vi "Stepper Sequence Change Focus.vi"() -> ()   [LabVIEW 2013]
doc: "Writes specified digital values to all 14 digital I/O pins. Each pin must first be configured as a digital output using the Arduino Set Digital Pin Mode VI."
uses:
  Hello Optotune Lens (30.06.2014)/Calibration.ctl
  <vilib>/Math Plots/3D Math Plots/3D Surface/3D Surface XCtrl/3D Surface.xctl
  <vilib>/LabVIEW Interface for Arduino/Type Defs/Board Type.ctl
  <vilib>/LabVIEW Interface for Arduino/Type Defs/Analog Pin.ctl
  <vilib>/Instr/_visa.llb/VISA Configure Serial Port (Instr).vi
  <vilib>/Math Plots/3D Math Plots/3D Surface/3D Surface Datatype/Public/Plot Helper (Matrix).vi
  <vilib>/LabVIEW Interface for Arduino/LabVIEW Interface for Arduino.lvlib
  <vilib>/Math Plots/3D Math Plots/3D Surface/3D Surface Datatype/3D Surface Datatype.lvclass
panel:
  out "3D Surface":refnum<class "3D Plot Datatype.lvclass">[](xcontrol)
  in  "Anahl Messungen":i32
  out "Aktuelle Messung":i32
  in  "Maximaler Strom":dbl=290.0
  out "Array 2":dbl[](array[numeric])
  out "Voltage 2":dbl(knob)=0.0294 scale=0.0..5.0
  in  "Stepwidth X":dbl=20.0
  out "Array":dbl[](array[numeric])=[0.0784, 0.0, 0.0, 0.0, 0.049, 0.053899999999999997, 0.0784, 0.0392, 0.0588, 0.0294]
  out "Aktueller Linsenstrom":dbl=49.0
  out "Schritt 7":bool
  out "Schritt 6":bool
  out "Schritt 5":bool
  out "Schritt 4":bool
  out "Schritt 3":bool
  out "Schritt 2":bool
  out "Schritt 1":bool=TRUE
  out "Value":u8
  out "x = y?":bool=TRUE
  in  "STOP INTIAL":bool
  out "VISA resource name out 3":refnum<visa-resource-name>="COM13"
  out "Command to Port 2":string="Aw\n´"
  out "Number of Measurements":i8=6
  in  "Min Focal Length 2":dbl
  in  "Max Focal Length":dbl=293.0
  out "Position_aktuell":dbl=90.0
  in  "First Motor Pin":u8=3
  in  "Pin Endlagenschalter":u8=32
  in  "Stepwidth Focalwidth lens":dbl=50.0
  in  "Calibration":T1={"Max Current A"=293.0, "Max Current B"=293.0, "UCL A"=300.0, "UCL B"=300.0, "LCL A"=0.0, "LCL B"=0.0} {"Max Current A" format="%#_g mA"; "Max Current B" format="%#_g mA"; "UCL A" format="%#_g mA"; "LCL A" format="%#_g mA"; "UCL B" format="%#_g mA"; "LCL B" format="%#_g mA"}
  out "ID":u16
  out "VISA resource name out":string="COM13"
  out "Calibration 2":T1={"Max Current A"=292.84, "Max Current B"=293.0, "UCL A"=292.76850585937495, "UCL B"=300.0, "LCL A"=4392.671494140624, "LCL B"=0.0} {"Max Current A" format="%#_g mA"; "Max Current B" format="%#_g mA"; "UCL A" format="%#_g mA"; "LCL A" format="%#_g mA"; "UCL B" format="%#_g mA"; "LCL B" format="%#_g mA"}
  out "OK":bool=TRUE
  out "Data":string
  out "Command to Port":string
  out "TA (°C)":dbl=32.125
  out "error out":errorcluster={"status"=FALSE, "code"=1073676294, "source"="VISA Read in write read Lens Driver.vi->Stepper Sequence Change Focus.vi"}
  in  "error in (no error)":errorcluster
  in  "VISA resource name":string="COM13"
  in  "Initial Speed":dbl=1.0
  # "Lens Settings"
  # "Measurement Settings"
  # "Initial Settings"
  # "mA"
  # "0 Fast, 100 slow"
  # "mA"
  # "Diodenstrom I0"
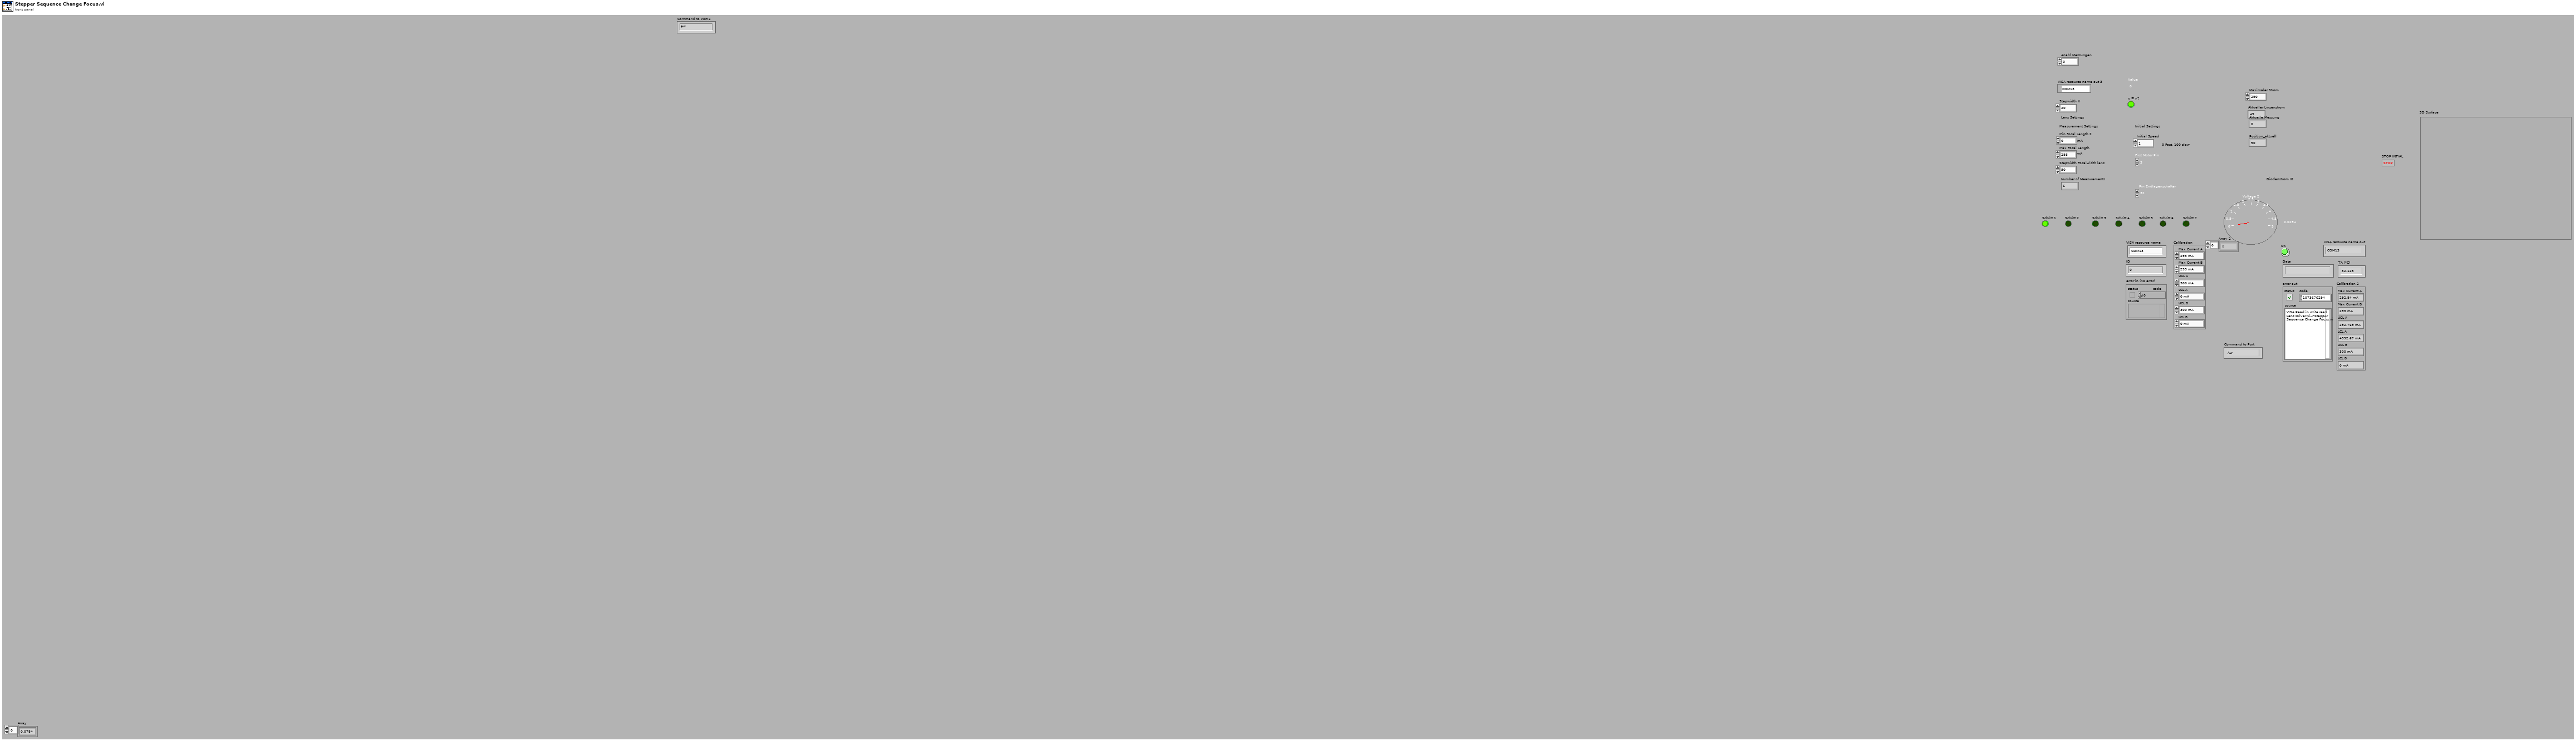
[diagram p1: front panel]
types:
  T1 = typedef "Calibration.ctl" = cluster{"Max Current A":dbl, "Max Current B":dbl, "UCL A":dbl, "UCL B":dbl, "LCL A":dbl, "LCL B":dbl}
  T2 = typedef "LabVIEW Interface for Arduino.lvlib/Board Type.ctl" = enum16{"Uno", "Dimuelanove w/Atmega 328", "Mega 2560"}
  T3 = typedef "LabVIEW Interface for Arduino.lvlib/Arduino Resource.ctl" = cluster{"VISA resource":refnum<visa-resource-name>, "Board Type":T2, "Connection Type":enum8{"USB / Serial"}, "Bytes Per Packet (15)":u8}
  T4 = typedef "LabVIEW Interface for Arduino.lvlib/Analog Pin.ctl" = enum8{"Anlog In 0", "Anlog In 1", "Anlog In 2", "Anlog In 3", "Anlog In 4", "Anlog In 5"}
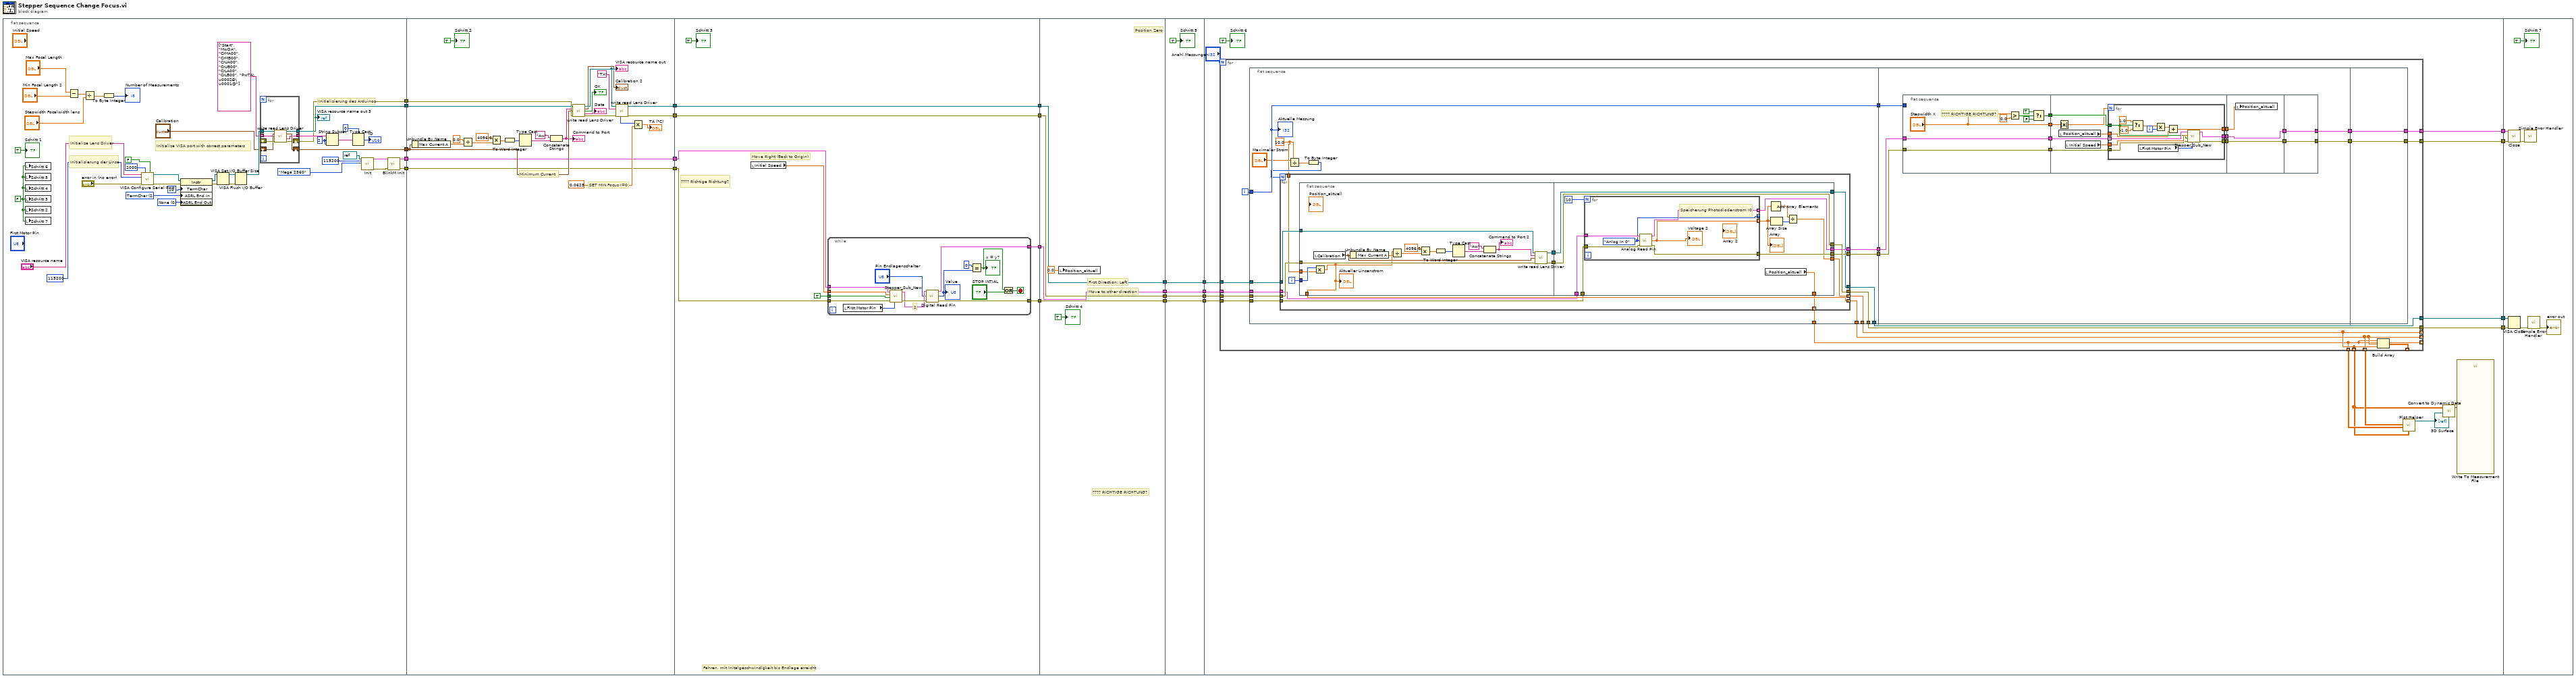
[diagram p0: block diagram]
diagram:
  n1 = flat-sequence {
    tunnel: [w43] -> w15
    tunnel: [w42] -> w14
    tunnel: [w41] -> w13
    tunnel: [w36] -> w5
    tunnel: [w35] -> w4
    tunnel: [w77] -> w25
    tunnel: [w76] -> w24
    tunnel: w15 -> [w99]
    tunnel: w14 -> [w98]
    tunnel: w13 -> [w97]
    tunnel: [w94] -> w12
    tunnel: [w78] -> w6
    tunnel: w5 -> [w77]
    tunnel: w4 -> [w76]
    tunnel: [w107] -> w19
    tunnel: w25 -> [w105]
    tunnel: [w106] -> w17
    tunnel: w24 -> [w108]
    tunnel: w12 -> [w104]
    tunnel: [w104] -> w11
    tunnel: [w103] -> w7
    tunnel: w6 -> [w103]
    tunnel: w19 -> [w129]
    tunnel: [w129] -> w18
    tunnel: w17 -> [w128]
    tunnel: [w128] -> w16
    tunnel: w11 -> [w127]
    tunnel: [w127] -> w10
    tunnel: [w126] -> w8
    tunnel: w7 -> [w126]
    tunnel: w18 -> [w133]
    tunnel: [w133] -> w23
    tunnel: w16 -> [w130]
    tunnel: [w130] -> w22
    tunnel: w10 -> [w132]
    tunnel: w8 -> [w131]
    tunnel: [w132] -> w3
    tunnel: [w131] -> w2
    tunnel: w23 -> [w149]
    tunnel: w22 -> [w148]
    tunnel: [w147] -> w21
    tunnel: [w146] -> w20
    tunnel: [w144] -> w9
    tunnel: w3 -> [w145]
    tunnel: w2 -> [w143]
    tunnel: [w141] -> w1
    tunnel: w21 -> [w290]
    tunnel: w20 -> [w289]
    tunnel: w9 -> [w286]
    tunnel: w1 -> [w287]
    frame #0 {
      w27 = FALSE ("Schritt 6")
      w63 = 2 ("length (rest)")
      w48 = u16 0 items=["None", "Last Bit", "TermChar", "Break"] ("Serial Settings:End Mode for Writes")
      w49 = u16 2 items=["None", "Last Bit", "TermChar"] ("Serial Settings:End Mode for Reads")
      # "Initialisierung des Arduinos"
      # "Initialisierung der Linse"
      # "Initialize Lens Driver"
      # "Initialize VISA port with correct parameters"
      n2 = local write "Schritt 6"(w27) -> ()
      n3 = local write "Schritt 5"(w27) -> ()
      n4 = local write "Schritt 4"(w27) -> ()
      n5 = local write "Schritt 3"(w27) -> ()
      n6 = local write "Schritt 2"(w27) -> ()
      n7 = local write "Schritt 7"(w27) -> ()
      n8 = Subtract(x="Max Focal Length", y="Min Focal Length 2") -> (x-y=w32:dbl)
      n9 = Divide(x=w32, y="Stepwidth Focalwidth lens") -> (x/y=w30:dbl)
      n10 = To Byte Integer(number=w30) -> (8bit integer=→"Number of Measurements":i8)
      n11 = call-poly "VISA Configure Serial Port"("VISA resource name"="VISA resource name", "timeout (10sec)"=u32 2000, "Enable Termination\nChar (T)"=FALSE ("Enable Termination\nChar (T)"), "baud rate (9600)"=u32 115200, "error in (no error)"="error in (no error)") -> ("VISA resource name out"=w53:refnum<visa-resource-name>, "error out"=w51:errorcluster)  [unwired: 9 in]
      n12 = property class="Instr"(reference=w53, error in=w51, "TermChar"=u8 10 ("Message Based Settings:Termination Character"), "ASRL End In"=w49, "ASRL End Out"=w48) -> (reference out=w52:refnum<visa-resource-name>, error out=w50:errorcluster)
      n13 = VISA Set I/O Buffer Size(VISA resource name=w52, error in (no error)=w50) -> (VISA resource name out=w45:refnum<visa-resource-name>, error out=w44:errorcluster)  [unwired: 2 in]
      n14 = VISA Flush I/O Buffer(VISA resource name=w45, error in (no error)=w44) -> (VISA resource name out=w65:refnum<visa-resource-name>)  [unwired: 1 in, 1 out]
      n15 = for {
        tunnel: w65 -> [w72]
        tunnel: [w69] -> w43
        tunnel: string[] ["Start", "MwDA", "CrMA00", "CrMB00", "CrUA00", "CrUB00", "CrLA00", "CrLB00", "PwTA\u0002Ð\u0001@"] -> [w67] mode=indexing
        tunnel: [w66] -> w59
        shift-right: [w70] -> w42
        shift-left: "Calibration" -> [w71]
        shift-right: [w68] -> w41
        shift-left: _ -> [w73]
        n16 = call "write read Lens Driver.vi"("VISA resource name"=w72, "command"=w67, "Calibration"=w71, "error in (no error)"=w73) -> ("VISA resource name out"=w69:refnum<visa-resource-name>, "Calibration 2"=w70:T1, "Data"=w66:string, "error out"=w68:errorcluster)  [unwired: 4 in, 4 out]
      }
      "VISA resource name out 3" <- w43
      n17 = String Subset(string=w59, offset (0)=w63, length (rest)=w63) -> (substring=w61:string)
      n18 = Type Cast(type=u16 0 ("length (rest)"), x=w61) -> (*(type *) &x=→"ID":u16)
      n19 = call <vilib>:"Init.vi"("VISA resource"=refnum<visa-resource-name> refnum, "Baud Rate (115200)"=u32 115200, "Board Type (Uno)"=Board_Type."Mega 2560") -> ("Arduino Resource"=w39:T3, "error out"=w40:errorcluster)  [unwired: 15 in]
      n20 = call <vilib>:"BlinkM Init.vi"("Arduino Resource"=w39, "error in"=w40) -> ("Arduino Resource"=w36:T3, "error out"=w35:errorcluster)  [unwired: 12 in]
      "Schritt 1" <- TRUE
    }
    frame #1 {
      # "Minimum Current"
      # "SET MIN Focus I=0"
      n21 = Unbundle By Name(w98) -> ("Max Current A"=w83:dbl)
      n22 = Divide(x=0.0, y=w83) -> (x/y=w90:dbl)
      n23 = Multiply(x=4096.0, y=w90) -> (x*y=w88:dbl)
      n24 = To Word Integer(number=w88) -> (16bit integer=w87:i16)
      n25 = Type Cast(x=w87) -> (*(type *) &x=w86:string)  [unwired: 1 in]
      n26 = Concatenate Strings("Aw", w86) -> (w84:string)
      "Command to Port" <- w84
      n27 = call "write read Lens Driver.vi"("VISA resource name"=w99, "command"=w84, "Calibration"=w98, "error in (no error)"=w97) -> ("VISA resource name out"=w96:refnum<visa-resource-name>, "Calibration 2"=→"Calibration 2":T1, "OK"=→"OK":bool, "Data"=→"Data":string, "error out"=w95:errorcluster)  [unwired: 4 in, 3 out]
      "VISA resource name out" <- w96
      n28 = call "write read Lens Driver.vi"("VISA resource name"=w96, "command"="TA", "error in (no error)"=w95) -> ("VISA resource name out"=w94:refnum<visa-resource-name>, "TA"=w80:u16, "error out"=w78:errorcluster)  [unwired: 5 in, 5 out]
      n29 = Multiply(x=w80, y=0.0625) -> (x*y=→"TA (°C)":dbl)
      "Schritt 2" <- TRUE
    }
    frame #2 {
      # "???? Richtige Richtung?"
      # "Move Right (Back to Origin)"
      # "Fahren, mit Initalgeschwindigkeit bis Endlage erreicht"
      n30 = local read "Initial Speed"() -> (w102:dbl)
      n31 = while {
        tunnel: w105 -> [w122]
        tunnel: w108 -> [w121]
        tunnel: TRUE -> [w119]
        tunnel: w102 -> [w120]
        tunnel: [w114] -> w107
        tunnel: [w113] -> w106
        stop <- w116 stop-if-true
        # "2"
        n32 = local read "First Motor Pin"() -> (w118:u8)
        n33 = call "Stepper_Sub_New.vi"("First Motor Pin"=w118, "error in"=w121, "Direction"=w119, "Velocity"=w120, "Arduino Resource"=w122) -> ("error out"=w111:errorcluster, "Arduino Resource 2"=w110:T3)  [unwired: 5 in]
        n34 = call <vilib>:"Digital Read Pin.vi"("Arduino Resource"=w110, "Digital I/O Pin (0)"="Pin Endlagenschalter", "error in"=w111) -> ("Arduino Resource"=w114:T3, "Value"=w112:u8, "error out"=w113:errorcluster)  [unwired: 10 in]
        "Value" <- w112
        n35 = Equal?(x=u8 0, y=w112) -> (x = y?=w117:bool)
        "x = y?" <- w117
        n36 = Or(x=w117, y="STOP INTIAL") -> (x .or. y?=w116:bool)
      }
      "Schritt 3" <- TRUE
    }
    frame #3 {
      # "???? RICHTIGE RICHTUNG?"
      # "Move to other direction"
      # "First Direction: Left"
      # "Position Zero"
      n37 = local write "Position_aktuell"(0.0 ("Position_aktuell")) -> ()
      "Schritt 4" <- TRUE
    }
    frame #4 {
      "Schritt 5" <- TRUE
    }
    frame #5 {
      n38 = for {
        N: "Anahl Messungen" -> [_]
        tunnel: w149 -> [w167]
        tunnel: w148 -> [w166]
        tunnel: [w165] -> w147
        tunnel: [w164] -> w146
        tunnel: w145 -> [w162]
        tunnel: w143 -> [w161]
        tunnel: [w159] -> w144
        tunnel: [w151] -> _ mode=indexing
        tunnel: [w155] -> w141
        tunnel: [w152] -> _ mode=indexing
        tunnel: [w150] -> _ mode=indexing
        tunnel: [w153] -> _ mode=indexing
        tunnel: [w152] -> w136 mode=indexing
        tunnel: [w151] -> w138 mode=indexing
        tunnel: [w150] -> w137 mode=indexing
        i -> [w160]
        n39 = flat-sequence {
          tunnel: w167 -> [w179]
          tunnel: w166 -> [w177]
          tunnel: [w178] -> w163
          tunnel: w162 -> [w183]
          tunnel: w161 -> [w180]
          tunnel: w160 -> [w173]
          tunnel: [w182] -> w159
          tunnel: [w181] -> w151
          tunnel: [w176] -> w156
          tunnel: [w175] -> w155
          tunnel: [w174] -> w152
          tunnel: [w173] -> w154
          tunnel: [w169] -> w150
          tunnel: w163 -> [w246]
          tunnel: [w245] -> w158
          tunnel: [w244] -> w157
          tunnel: w156 -> [w243]
          tunnel: w154 -> [w242]
          tunnel: [w284] -> w164
          tunnel: [w285] -> w165
          tunnel: w158 -> [w285]
          tunnel: w157 -> [w284]
          frame #0 {
            w168 = 10.0 ("y")
            n40 = Divide(x="Maximaler Strom", y=w168) -> (x/y=w171:dbl)
            n41 = To Byte Integer(number=w171) -> (8bit integer=w170:i8)
            n42 = for {
              N: w170 -> [_]
              tunnel: w183 -> [w196]
              tunnel: [w195] -> w182
              tunnel: [w194] -> w181 mode=indexing
              tunnel: w180 -> [w193]
              tunnel: w179 -> [w192]
              tunnel: [w191] -> w178
              tunnel: w177 -> [w190]
              tunnel: [w189] -> w176
              tunnel: [w188] -> w175
              tunnel: [w186] -> w174 mode=indexing
              tunnel: [w185] -> w169 mode=indexing
              tunnel: w168 -> [w184]
              i -> [w187]
              n43 = flat-sequence {
                tunnel: w196 -> [w207]
                tunnel: w193 -> [w206]
                tunnel: [w200] -> w194
                tunnel: [w204] -> w198
                tunnel: [w203] -> w197
                tunnel: w187 -> [w201]
                tunnel: w184 -> [w199]
                tunnel: [w218] -> w195
                tunnel: w198 -> [w219]
                tunnel: w197 -> [w218]
                tunnel: w192 -> [w222]
                tunnel: w190 -> [w217]
                tunnel: [w221] -> w189
                tunnel: [w220] -> w191
                tunnel: [w219] -> w188
                tunnel: [w216] -> w186
                tunnel: [w215] -> w185
                frame #0 {
                  n44 = local read "Calibration"() -> (w202:T1)
                  n45 = Multiply(x=w201, y=w199) -> (x*y=w200:dbl)
                  "Aktueller Linsenstrom" <- w200
                  n46 = Unbundle By Name(w202) -> ("Max Current A"=w205:dbl)
                  n47 = Divide(x=w200, y=w205) -> (x/y=w214:dbl)
                  n48 = Multiply(x=4096.0, y=w214) -> (x*y=w212:dbl)
                  n49 = To Word Integer(number=w212) -> (16bit integer=w211:i16)
                  n50 = Type Cast(x=w211) -> (*(type *) &x=w210:string)  [unwired: 1 in]
                  n51 = Concatenate Strings("Aw", w210) -> (w208:string)
                  "Command to Port 2" <- w208
                  n52 = call "write read Lens Driver.vi"("VISA resource name"=w207, "command"=w208, "Calibration"=w202, "error in (no error)"=w206) -> ("VISA resource name out"=w204:refnum<visa-resource-name>, "error out"=w203:errorcluster)  [unwired: 4 in, 6 out]
                }
                frame #1 {
                  n53 = for {
                    N: 10 -> [_]
                    tunnel: w217 -> [w232]
                    tunnel: w222 -> [w231]
                    tunnel: [w230] -> w221 mode=indexing
                    tunnel: [w229] -> w220
                    tunnel: [w228] -> _ mode=indexing
                    tunnel: [w227] -> w223 mode=indexing
                    w228 = Analog_Pin."Anlog In 0" ("Photodiode Pin")
                    # "Speicherung Photodiodenstrom I0"
                    n54 = call <vilib>:"Analog Read Pin.vi"("Arduino Resource"=w231, "Analog Input Pin (0)"=w228, "error in"=w232) -> ("Arduino Resource"=w230:T3, "Voltage"=w227:dbl, "error out"=w229:errorcluster)  [unwired: 10 in]
                    "Voltage 2" <- w227
                  }
                  "Array" <- w223
                  n55 = local read "Position_aktuell"() -> (w215:dbl)
                  n56 = Add Array Elements(numeric array=w223) -> (sum=w224:dbl)
                  n57 = Array Size(array=w223) -> (size(s)=w225:i32)
                  n58 = Divide(x=w224, y=w225) -> (x/y=w216:dbl)
                }
              }
            }
            "Aktuelle Messung" <- w173
          }
          frame #1 {
            n59 = flat-sequence {
              tunnel: w246 -> [w248]
              tunnel: [w248] -> w241
              tunnel: ["Stepwidth X"] -> w240
              tunnel: [w250] -> w239
              tunnel: [w249] -> w238
              tunnel: w243 -> [w249]
              tunnel: w242 -> [_]
              tunnel: [w263] -> w236
              tunnel: [w262] -> w237
              tunnel: w241 -> [w264]
              tunnel: w240 -> [w259]
              tunnel: w239 -> [w260]
              tunnel: w238 -> [w257]
              tunnel: [w255] -> w235
              tunnel: w237 -> [w280]
              tunnel: w236 -> [w281]
              tunnel: [w281] -> w234
              tunnel: [w280] -> w233
              tunnel: w235 -> [w279]
              tunnel: [w282] -> w244
              tunnel: [w283] -> w245
              tunnel: w234 -> [w283]
              tunnel: w233 -> [w282]
              frame #0 {
                # "???? RICHTIGE RICHTUNG?"
                n60 = Greater?(x="Stepwidth X", y=0.0) -> (0:w253:bool)
                n61 = Select(t=TRUE, s=w253, f=FALSE) -> (s? t:f=w250:bool)
              }
              frame #1 {
                n62 = Absolute Value(x=w259) -> (abs(x)=w258:dbl)
                n63 = local read "Position_aktuell"() -> (w256:dbl)
                n64 = local read "Initial Speed"() -> (w261:dbl)
                n65 = for {
                  N: w258 -> [_]
                  tunnel: w264 -> [w273]
                  tunnel: [w276] -> w263
                  tunnel: [w275] -> w262
                  tunnel: w261 -> [w278]
                  tunnel: w260 -> [w272]
                  tunnel: w257 -> [w274] mode=indexing
                  tunnel: w256 -> [w266]
                  tunnel: [w265] -> w255
                  i -> [w268]
                  n66 = Select(t=1.0, s=w272, f=-1.0) -> (s? t:f=w269:dbl)
                  n67 = local read "First Motor Pin"() -> (w277:u8)
                  n68 = Multiply(x=w269, y=w268) -> (x*y=w267:dbl)
                  n69 = Add(x=w267, y=w266) -> (x+y=w265:dbl)
                  n70 = call "Stepper_Sub_New.vi"("First Motor Pin"=w277, "error in"=w273, "Direction"=w272, "Velocity"=w278, "Arduino Resource"=w274) -> ("error out"=w275:errorcluster, "Arduino Resource 2"=w276:T3)  [unwired: 5 in]
                }
              }
              frame #2 {
                n71 = local write "Position_aktuell"(w279) -> ()
              }
              frame #3 {
              }
            }
          }
          frame #2 {
          }
        }
        n72 = Build Array(w150, w151, w152) -> (w153:dbl[][])
      }
      n73 = call-poly <vilib>:"Plot Helper.vi"("z matrix"=w136, "y matrix"=w137, "x matrix"=w138) -> ("3D Plot lvclass Array out"=→"3D Surface":refnum<class "3D Plot Datatype.lvclass">[])  [unwired: 3 in, 5 out]
      n74 = call "Convert to Dynamic Data"("2D Array"=w136) -> ("Dynamic Data Type"=w135:dynamicdata)  [unwired: 3 in]
      n75 = call "Write To Measurement File"("Signals"=w135) -> ()  [unwired: 16 in, 3 out]
      "Schritt 6" <- TRUE
    }
    frame #6 {
      n76 = call <vilib>:"Close.vi"("Arduino Resource"=w290, "error in"=w289) -> ("error out"=w293:errorcluster)  [unwired: 13 in]
      n77 = VISA Close(VISA resource name=w287, error in (no error)=w286) -> (error out=w291:errorcluster)
      n78 = call <vilib>:"Simple Error Handler.vi"("error in (no error)"=w293) -> ()  [unwired: 4 in, 5 out]
      n79 = call <vilib>:"Simple Error Handler.vi"("error in (no error)"=w291) -> ("error out"=→"error out":errorcluster)  [unwired: 4 in, 4 out]
      "Schritt 7" <- TRUE
    }
  }
